vi "SignalMngmnt.vi"(8 "error in (no error)":errorcluster) -> (0 "error out":errorcluster)   [LabVIEW 2012]
uses:
  #TD_SignalStorageCommand.ctl
  #TD_SignalStorageData.ctl
  <vilib>/addons/Wavelet Analysis/typedefs.llb/WA Data.ctl
  <vilib>/Waveform/WDTOps.llb/WDT Get Waveform Subset DBL.vi
  <vilib>/addons/_Advanced Signal Processing/NI_AdvSigProcWA.lvlib
panel:
  in  "CursorReset":bool
  in  "ResetStorage":bool
  in  "Cut":bool
  out "Signal Graph":waveform(dbl)(graph) caption="Podgląd sygnału"
  in  "Signal Description":string caption="Opis sygnału"
  in  "Signal name":string caption="Nazwa sygnału:"
  in  "AddSpecial":bool
  in  "Remove":bool
  in  "Read":bool
  in  "Signal List":i32(listbox) caption="Lista sygnałów"
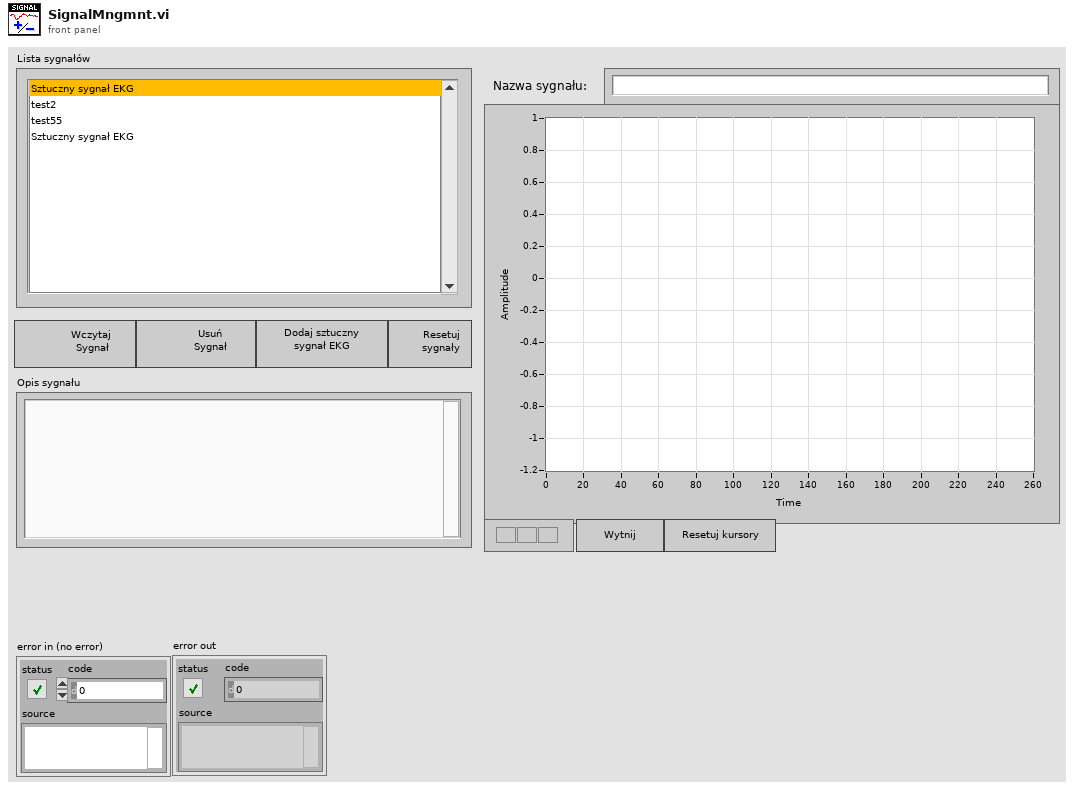
[diagram p1: front panel]
types:
  T1 = cluster{"Signal List":refnum<vi>, "Signal Graph":refnum<vi>, "Signal name":refnum<vi>, "Signal Description":refnum<vi>}
  T2 = typedef "#TD_SignalStorageCommand.ctl" = enum16{"Reset_Storage", "Add_Signal", "Insert_Signal", "Del_Signal", "Replace_Signal", "Get_Signal", "Get_Signal_List", "Change_Signal_Name", "Change_Signal_Descr"}
  T3 = typedef "#TD_SignalStorageData.ctl" = cluster{"Signal":waveform(dbl), "Signal Name":string, "Description":string}
  T4 = typedef "#TD_SignalSpecInfo.ctl" = cluster{"file name":string, "format":i32, "samples per frame":i32, "skew":i32, "byte offset":i32, "ADC gain":dbl, "baseline (ADC units)":i16, "units":string, "ADC resolution":i16, "ADC zero":i16, "initial value":i16, "checksum":i16, "block size":i32, "description":string}
  T5 = typedef "NI_AdvSigProcWA.lvlib/WA Data.ctl" = u16
  T6 = typedef "LVPoint32TypeDef.ctl" = cluster{"Horizontal":i32, "Vertical":i32}
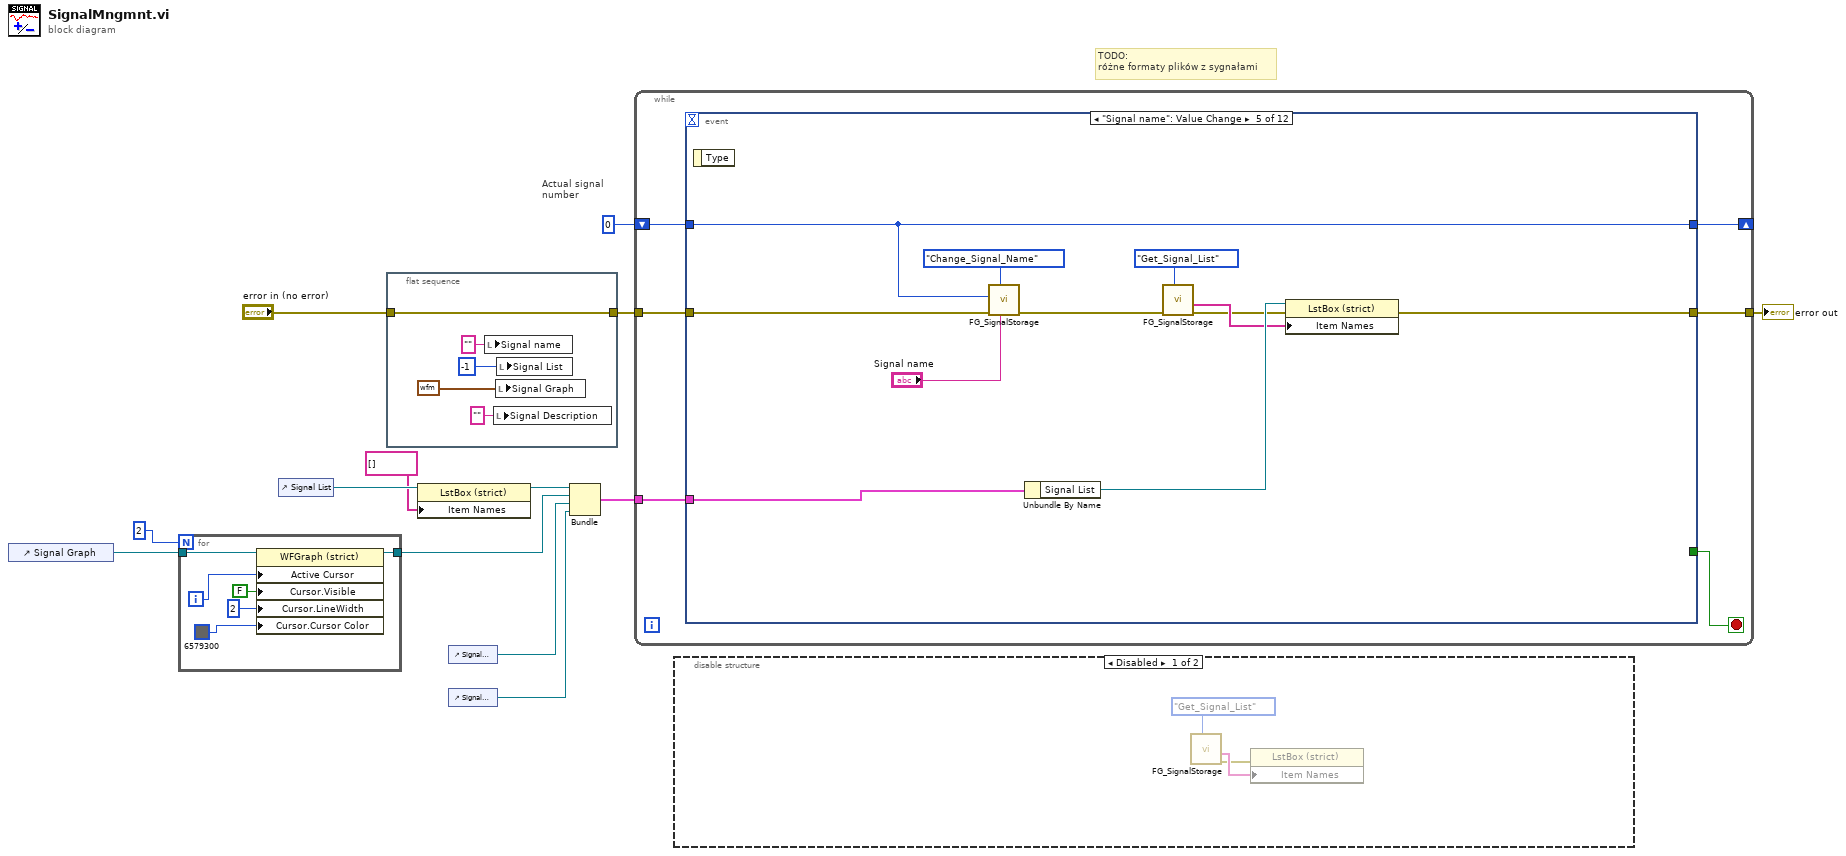
[diagram p0: block diagram]
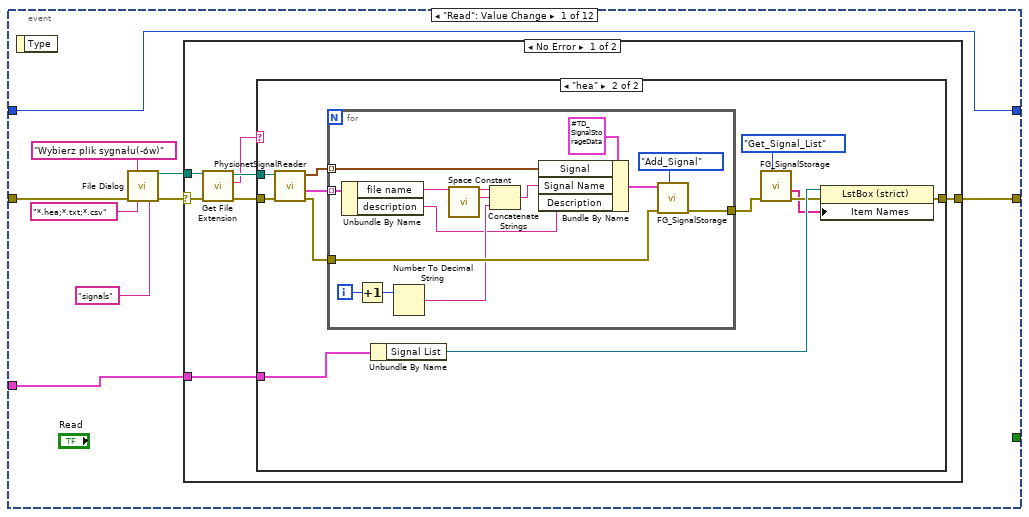
[diagram p3: hidden frame]
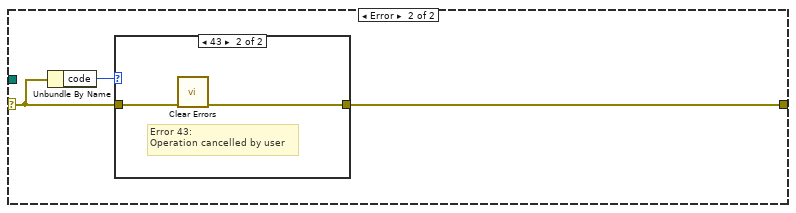
[diagram p5: hidden frame]
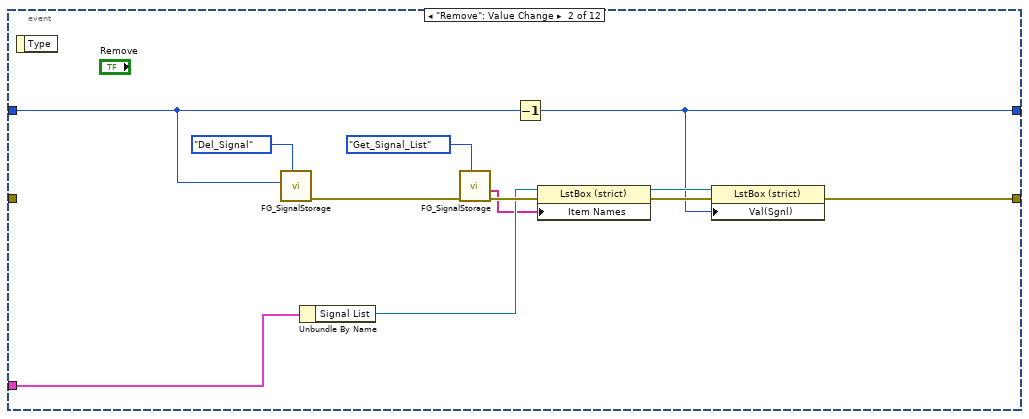
[diagram p7: hidden frame]
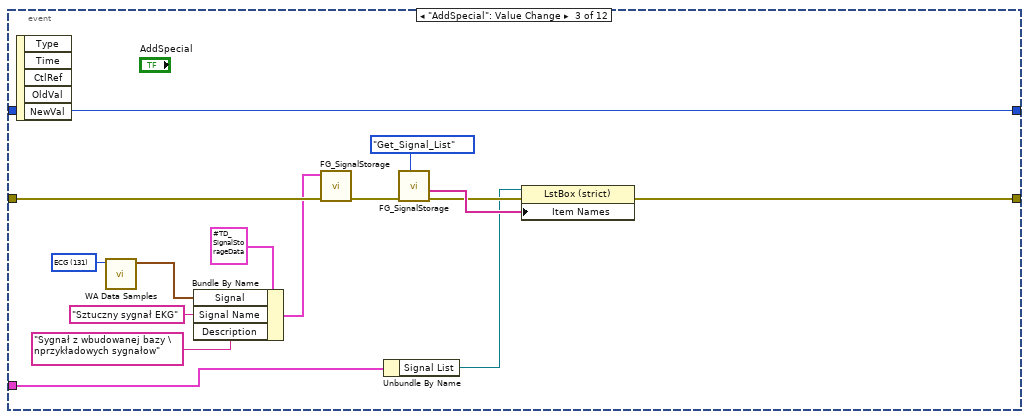
[diagram p8: hidden frame]
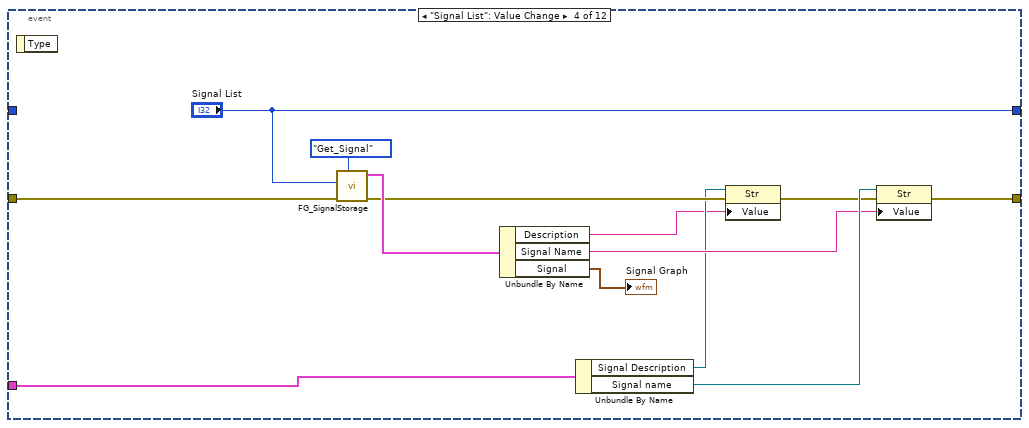
[diagram p9: hidden frame]
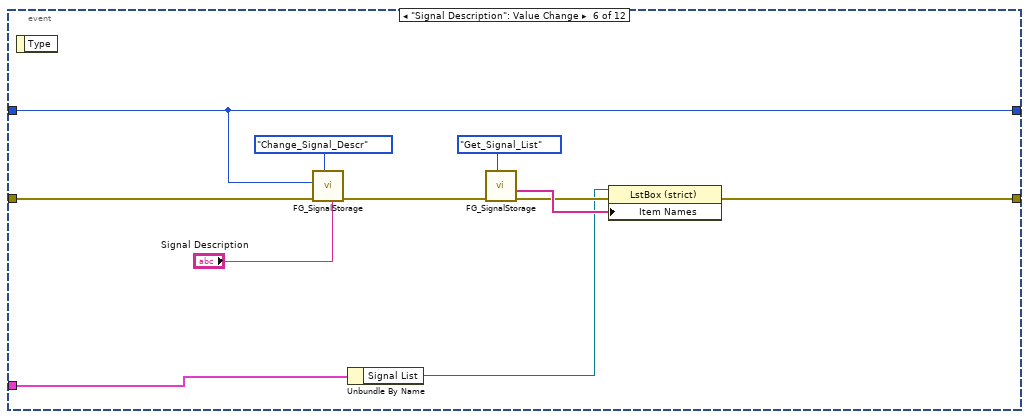
[diagram p10: hidden frame]
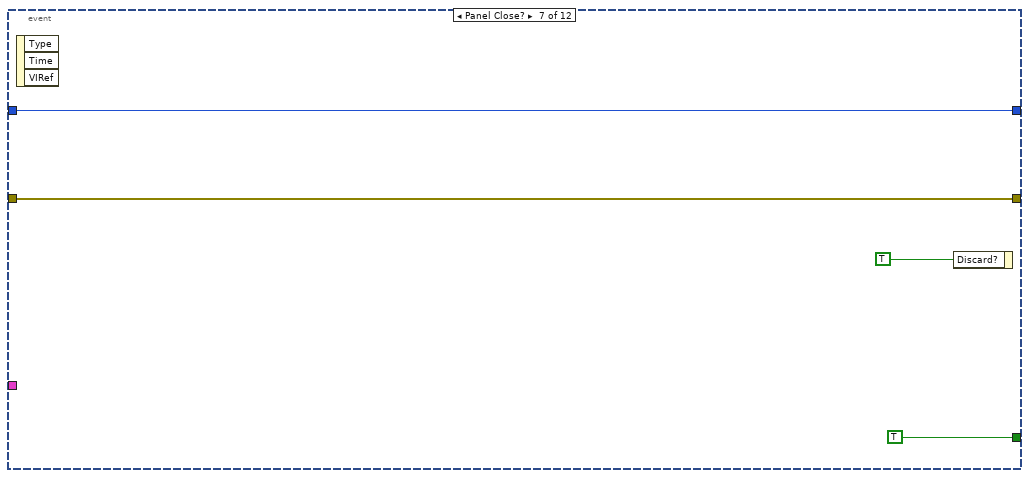
[diagram p11: hidden frame]
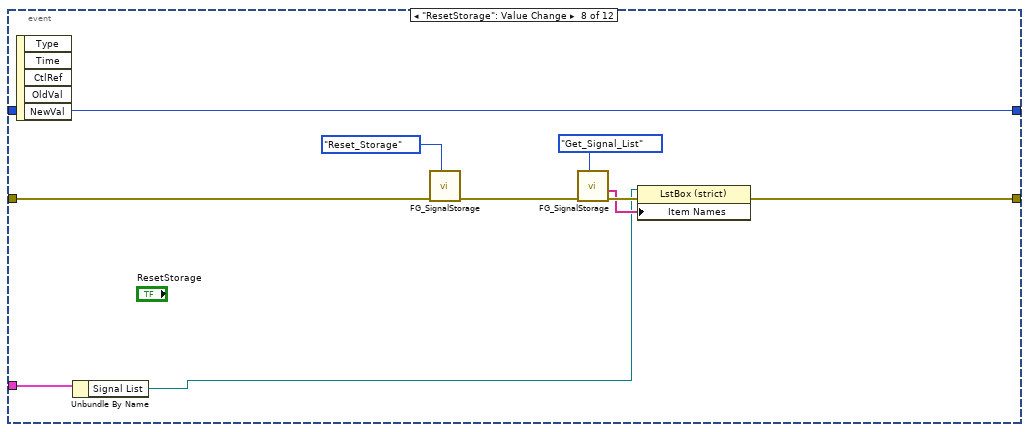
[diagram p12: hidden frame]
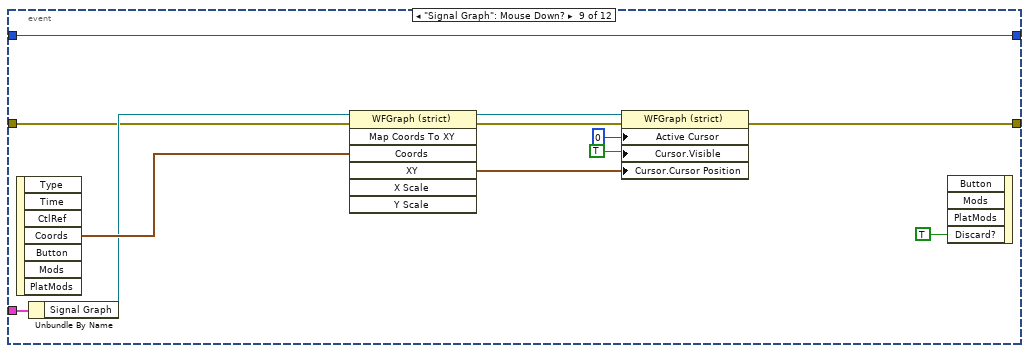
[diagram p13: hidden frame]
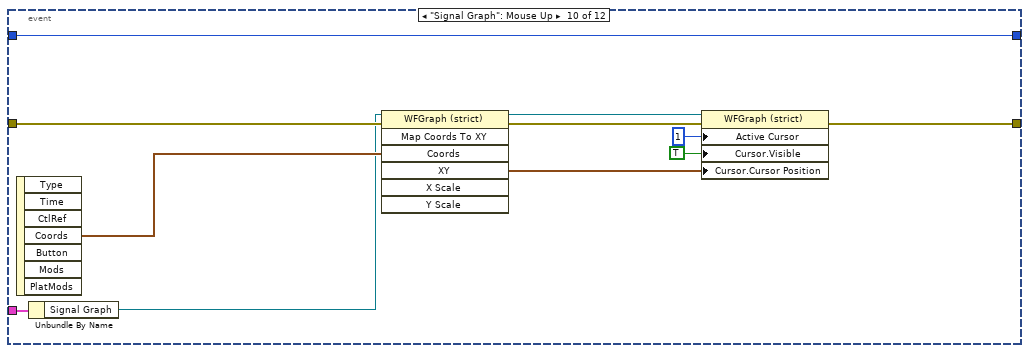
[diagram p14: hidden frame]
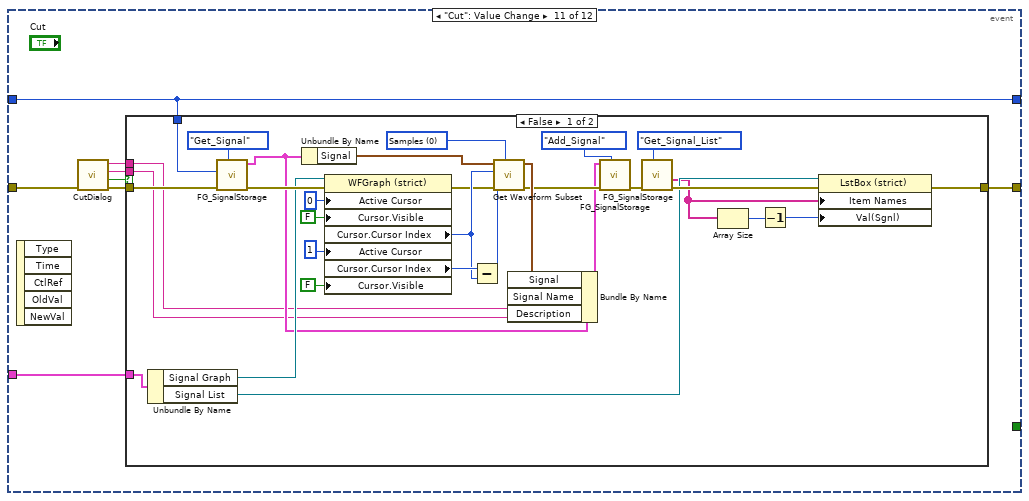
[diagram p15: hidden frame]
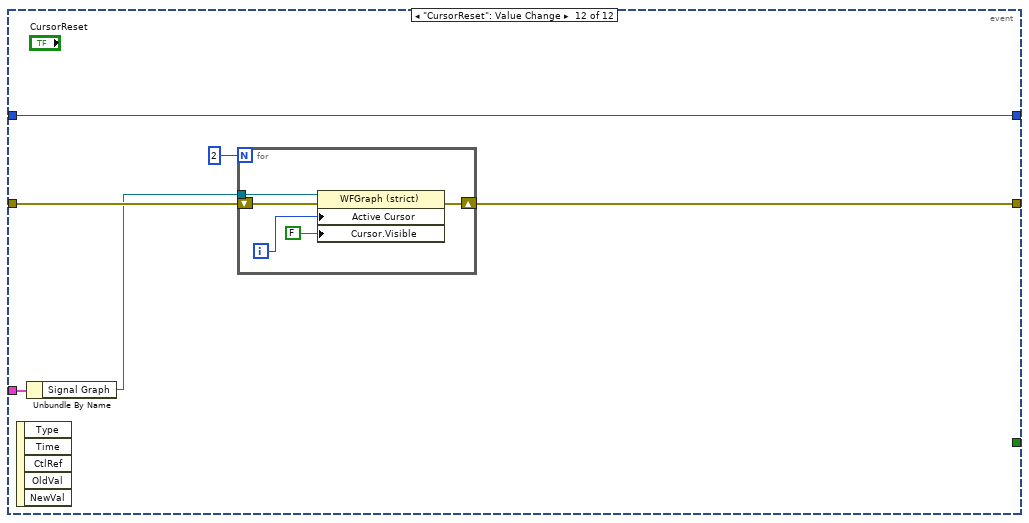
[diagram p17: hidden frame]
diagram:
  # "Actual signal\nnumber"
  # "TODO:\nróżne formaty plików z sygnałami"
  n1 = control-ref of="Signal Graph"() -> (w5:refnum<vi>)
  n2 = for {
    N: 2 -> [_]
    tunnel: w5 -> [w17]
    tunnel: [w16] -> w4
    i -> [w19]
    n3 = property class="WFGraph (strict)"(reference=w17, "Active Cursor"=w19, "Cursor.Visible"=FALSE, "Cursor.LineWidth"=u8 2 ("Cursor.Line Width"), "Cursor.Cursor Color"=u32 6579300) -> (reference out=w16:refnum<vi>)  [unwired: 1 in, 1 out]
  }
  n4 = control-ref of="Signal List"() -> (w11:refnum<vi>)
  n5 = flat-sequence {
    tunnel: [w20] -> w3
    tunnel: "error in (no error)" -> [w20]
    frame #0 {
      n6 = local write "Signal name"("" ("Signal name")) -> ()
      n7 = local write "Signal Description"("" ("Signal Description")) -> ()
      n8 = local write "Signal Graph"(waveform(dbl) {"t0"=timestamp(0 s since 1904-01-01), "dt"=0.0, "Y"=[]} ("Podgląd sygnału")) -> ()
      n9 = local write "Signal List"(-1 ("Lista sygnałów")) -> ()
    }
  }
  n10 = property class="LstBox (strict)"(reference=w11, "Item Names"=string[] []) -> (reference out=w10:refnum<vi>)  [unwired: 1 in, 1 out]
  n11 = control-ref of="Signal name"() -> (w8:refnum<vi>)
  n12 = control-ref of="Signal Description"() -> (w7:refnum<vi>)
  n13 = Bundle("Signal List"=w10, "Signal Graph"=w4, "Signal name"=w8, "Signal Description"=w7) -> (w13:T1)  [unwired: 1 in]
  n14 = while {
    tunnel: [w29] -> w1
    tunnel: w13 -> [w28]
    shift-right: [w26] -> _
    shift-left: 0 ("Lista sygnałów") -> [w27]
    tunnel: w3 -> [w25]
    stop <- w30 stop-if-true
    n15 = event shown="[4] \"Signal name\": Value Change" {
      selector: _ -> [_ _ _ _ _ _ _ _ _ _ _ _]
      dyn-events: _ -> [_ _ _ _ _ _ _ _ _ _ _ _]
      timeout: _ -> [_ _ _ _ _ _ _ _ _ _ _ _]
      tunnel: [_ _ _ _ _ _ TRUE _ _ _ _ _] -> w30
      tunnel: [w34 w83 w96 w112 w127 w133 w142 w148 w156 w168 w181 w220] -> w29
      tunnel: w28 -> [w33 w87 w94 w116 w126 w132 _ w147 w165 w177 w179 w222]
      tunnel: w27 -> [w32 w82 w106 _ w124 w138 w144 w155 w167 w178 w180 w224]
      tunnel: [w32 w80 w106 "Signal List" w124 w138 w144 w155 w167 w178 w180 w224] -> w26
      tunnel: w25 -> [w31 _ w104 w111 w129 w141 w142 w153 w159 w173 w186 w223]
      event "Read": Value Change {
        n16 = event-data() -> ()  [unwired: 1 in, 1 out]
        n17 = call "File Dialog"("prompt"="Wybierz plik sygnału(-ów)", "error in"=w31, "pattern (all files)"="*.hea;*.txt;*.csv", "pattern label"="signals") -> ("selected path"=w37:path, "error out"=w36:errorcluster)  [unwired: 8 in, 2 out]
        n18 = case shown="No Error" w36 {
          selector: w36 -> [w44 w75]
          tunnel: w37 -> [w46 _]
          tunnel: [w41 w74] -> w34
          tunnel: w33 -> [w40 _]
          frame No Error {
            n19 = call <vilib>:"Get File Extension.vi"("error in (no error)"=w44, "file"=w46) -> ("error out"=w43:errorcluster, "lowercase file extension"=w42:string, "dup file"=w45:path)  [unwired: 6 in, 1 out]
            n20 = case shown="\"hea\"" w42 {
              tunnel: w45 -> [_ w57]
              tunnel: w43 -> [w47 w56]
              tunnel: [w47 w49] -> w41
              tunnel: w40 -> [_ w51]
              frame Default {
              }
              frame "hea" {
                n21 = call "PhysionetSignalReader.vi"("error in (no error)"=w56, "Header file path"=w57) -> ("error out"=w55:errorcluster, "Signals Specs Info"=w59:T4[], "Signals(physical units)"=w58:waveform(dbl)[])  [unwired: 5 in, 2 out]
                n22 = for {
                  tunnel: w59 -> [w73] mode=indexing
                  tunnel: w58 -> [w66] mode=indexing
                  tunnel: w55 -> [w64]
                  tunnel: [w63] -> w53
                  i -> [w72]
                  n23 = Unbundle By Name(w73) -> ("file name"=w70:string, "description"=w60:string)
                  n24 = Increment(x=w72) -> (x+1=w71:i32)
                  n25 = Number To Decimal String(number=w71) -> (decimal integer string=w62:string)  [unwired: 1 in]
                  n26 = call <vilib>:"Space Constant.vi"() -> ("String"=w61:string)
                  n27 = Concatenate Strings(w70, w61, w62) -> (w68:string)
                  n28 = Bundle By Name(cluster=T3 {"Signal"={"t0"=timestamp(0 s since 1904-01-01), "dt"=1.0, "Y"=[]}, "Signal Name"="", "Description"=""} ("DataIn"), "Signal"=w66, "Signal Name"=w68, "Description"=w60) -> (w65:T3)
                  n29 = call "FG_SignalStorage.vi"("Command"=#TD_SignalStorageCommand."Add_Signal", "error in (no error)"=w64, "DataIn"=w65) -> ("error out"=w63:errorcluster)  [unwired: 6 in, 2 out]
                }
                n30 = Unbundle By Name(w51) -> ("Signal List"=w52:refnum<vi>)
                n31 = call "FG_SignalStorage.vi"("Command"=#TD_SignalStorageCommand."Get_Signal_List", "error in (no error)"=w53) -> ("error out"=w50:errorcluster, "Signal_List"=w48:string[])  [unwired: 7 in, 1 out]
                n32 = property class="LstBox (strict)"(reference=w52, error in=w50, "Item Names"=w48) -> (error out=w49:errorcluster)  [unwired: 1 out]
              }
            }
          }
          frame Error {
            n33 = Unbundle By Name(w75) -> ("code"=w76:i32)
            n34 = case shown="43" w76 {
              tunnel: w75 -> [w77 w79]
              tunnel: [w77 w78] -> w74
              frame Default {
              }
              frame 43 {
                # "Error 43: \nOperation cancelled by user"
                n35 = call <vilib>:"Clear Errors.vi"("error in (no error)"=w79) -> ("error out"=w78:errorcluster)  [unwired: 6 in]
              }
            }
          }
        }
      }
      event "Remove": Value Change {
        n36 = event-data() -> ()  [unwired: 1 in, 1 out]
        n37 = call "FG_SignalStorage.vi"("Command"=#TD_SignalStorageCommand."Del_Signal", "SignalNumber"=w82) -> ("error out"=w88:errorcluster)  [unwired: 7 in, 2 out]
        n38 = Unbundle By Name(w87) -> ("Signal List"=w86:refnum<vi>)
        n39 = call "FG_SignalStorage.vi"("Command"=#TD_SignalStorageCommand."Get_Signal_List", "error in (no error)"=w88) -> ("error out"=w90:errorcluster, "Signal_List"=w81:string[])  [unwired: 7 in, 1 out]
        n40 = Decrement(x=w82) -> (x-1=w80:i32)
        n41 = property class="LstBox (strict)"(reference=w86, error in=w90, "Item Names"=w81) -> (reference out=w84:refnum<vi>, error out=w85:errorcluster)
        n42 = property class="LstBox (strict)"(reference=w84, error in=w85, "Val(Sgnl)"=w80) -> (error out=w83:errorcluster)  [unwired: 1 out]
      }
      event "AddSpecial": Value Change {
        w105 = T5 131 items=["1D Example Data"=100, "-"=101, "Doppler"=102, "HOP"=103, "TF Sine"=104, "Noisy Doppler"=105, "Sea Temperature"=106, "Sp500"=107, "Power Line"=108, "Engine Knocking"=109, "HeaviSine"=110, "Bumps"=111, "Blocks"=112, "Piece Regular"=113, "HypChirps"=114, "LinChirps"=115, "Chirps"=116, "Piece Polynomial"=117, "ECG"=131, "-"=118, "2D Example Data"=119, "-"=120, "Finger Print (Image)"=121, "Iris Flower (Image)"=122, "Mammogram (Image)"=123, "Lake (Image)"=127, "Two Can 1 (Image)"=132, "Two Can 2 (Image)"=133, "Camera Man (Image)"=134] ("data")
        n43 = event-data() -> ()  [unwired: 1 in, 5 out]
        n44 = call <vilib>:"WA Data Samples.vi"("data"=w105) -> ("signal"=w102:waveform(dbl))  [unwired: 9 in, 1 out]
        n45 = Bundle By Name(cluster=T3 {"Signal"={"t0"=timestamp(0 s since 1904-01-01), "dt"=1.0, "Y"=[]}, "Signal Name"="", "Description"=""} ("DataIn"), "Signal"=w102, "Signal Name"="Sztuczny sygnał EKG", "Description"="Sygnał z wbudowanej bazy \nprzykładowych sygnałow") -> (w101:T3)
        n46 = call "FG_SignalStorage.vi"("error in (no error)"=w104, "DataIn"=w101) -> ("error out"=w97:errorcluster)  [unwired: 7 in, 2 out]
        n47 = Unbundle By Name(w94) -> ("Signal List"=w93:refnum<vi>)
        n48 = call "FG_SignalStorage.vi"("Command"=#TD_SignalStorageCommand."Get_Signal_List", "error in (no error)"=w97) -> ("error out"=w98:errorcluster, "Signal_List"=w99:string[])  [unwired: 7 in, 1 out]
        n49 = property class="LstBox (strict)"(reference=w93, error in=w98, "Item Names"=w99) -> (error out=w96:errorcluster)  [unwired: 1 out]
      }
      event "Signal List": Value Change {
        n50 = event-data() -> ()  [unwired: 1 in, 1 out]
        n51 = call "FG_SignalStorage.vi"("Command"=#TD_SignalStorageCommand."Get_Signal", "error in (no error)"=w111, "SignalNumber"="Signal List") -> ("error out"=w110:errorcluster, "DataOut"=w117:T3)  [unwired: 6 in, 1 out]
        n52 = Unbundle By Name(w117) -> ("Description"=w107:string, "Signal Name"=w114:string, "Signal"=→"Signal Graph":waveform(dbl))
        n53 = Unbundle By Name(w116) -> ("Signal Description"=w109:refnum<vi>, "Signal name"=w115:refnum<vi>)
        n54 = property class="Str"(reference=w109, error in=w110, "Value"=w107) -> (error out=w108:errorcluster)  [unwired: 1 out]
        n55 = property class="Str"(reference=w115, error in=w108, "Value"=w114) -> (error out=w112:errorcluster)  [unwired: 1 out]
      }
      event "Signal name": Value Change {
        n56 = event-data() -> ()  [unwired: 1 in, 1 out]
        n57 = call "FG_SignalStorage.vi"("Signal Name"="Signal name", "Command"=#TD_SignalStorageCommand."Change_Signal_Name", "error in (no error)"=w129, "SignalNumber"=w124) -> ("error out"=w123:errorcluster)  [unwired: 5 in, 2 out]
        n58 = Unbundle By Name(w126) -> ("Signal List"=w125:refnum<vi>)
        n59 = call "FG_SignalStorage.vi"("Command"=#TD_SignalStorageCommand."Get_Signal_List", "error in (no error)"=w123) -> ("error out"=w120:errorcluster, "Signal_List"=w121:string[])  [unwired: 7 in, 1 out]
        n60 = property class="LstBox (strict)"(reference=w125, error in=w120, "Item Names"=w121) -> (error out=w127:errorcluster)  [unwired: 1 out]
      }
      event "Signal Description": Value Change {
        n61 = event-data() -> ()  [unwired: 1 in, 1 out]
        n62 = call "FG_SignalStorage.vi"("Signal Descr."="Signal Description", "Command"=#TD_SignalStorageCommand."Change_Signal_Descr", "error in (no error)"=w141, "SignalNumber"=w138) -> ("error out"=w134:errorcluster)  [unwired: 5 in, 2 out]
        n63 = Unbundle By Name(w132) -> ("Signal List"=w131:refnum<vi>)
        n64 = call "FG_SignalStorage.vi"("Command"=#TD_SignalStorageCommand."Get_Signal_List", "error in (no error)"=w134) -> ("error out"=w135:errorcluster, "Signal_List"=w136:string[])  [unwired: 7 in, 1 out]
        n65 = property class="LstBox (strict)"(reference=w131, error in=w135, "Item Names"=w136) -> (error out=w133:errorcluster)  [unwired: 1 out]
      }
      event Panel Close? {
        n66 = event-data() -> ()  [unwired: 1 in, 3 out]
        n67 = event-data("Discard?"=TRUE) -> ()  [unwired: 1 in, 1 out]
      }
      event "ResetStorage": Value Change {
        n68 = event-data() -> ()  [unwired: 1 in, 5 out]
        n69 = Unbundle By Name(w147) -> ("Signal List"=w146:refnum<vi>)
        n70 = call "FG_SignalStorage.vi"("Command"=#TD_SignalStorageCommand."Reset_Storage", "error in (no error)"=w153) -> ("error out"=w149:errorcluster)  [unwired: 7 in, 2 out]
        n71 = call "FG_SignalStorage.vi"("Command"=#TD_SignalStorageCommand."Get_Signal_List", "error in (no error)"=w149) -> ("error out"=w151:errorcluster, "Signal_List"=w150:string[])  [unwired: 7 in, 1 out]
        n72 = property class="LstBox (strict)"(reference=w146, error in=w151, "Item Names"=w150) -> (error out=w148:errorcluster)  [unwired: 1 out]
      }
      event "Signal Graph": Mouse Down? {
        n73 = event-data() -> ("Coords"=w162:T6)  [unwired: 1 in, 6 out]
        n74 = Unbundle By Name(w165) -> ("Signal Graph"=w161:refnum<vi>)
        n75 = invoke class="WFGraph (strict)" method="Map Coords To XY"(reference=w161, error in=w159, "Coords"=w162) -> (reference out=w160:refnum<vi>, error out=w158:errorcluster, "XY"=w157:cluster{"X":dbl, "Y":dbl})  [unwired: 4 in, 4 out]
        n76 = property class="WFGraph (strict)"(reference=w160, error in=w158, "Active Cursor"=u32 0, "Cursor.Visible"=TRUE, "Cursor.Cursor Position"=w157) -> (error out=w156:errorcluster)  [unwired: 1 out]
        n77 = event-data("Discard?"=TRUE) -> ()  [unwired: 4 in, 1 out]
      }
      event "Signal Graph": Mouse Up {
        n78 = event-data() -> ("Coords"=w174:T6)  [unwired: 1 in, 6 out]
        n79 = Unbundle By Name(w177) -> ("Signal Graph"=w170:refnum<vi>)
        n80 = invoke class="WFGraph (strict)" method="Map Coords To XY"(reference=w170, error in=w173, "Coords"=w174) -> (reference out=w169:refnum<vi>, error out=w171:errorcluster, "XY"=w172:cluster{"X":dbl, "Y":dbl})  [unwired: 4 in, 4 out]
        n81 = property class="WFGraph (strict)"(reference=w169, error in=w171, "Active Cursor"=u32 1, "Cursor.Visible"=TRUE, "Cursor.Cursor Position"=w172) -> (error out=w168:errorcluster)  [unwired: 1 out]
      }
      event "Cut": Value Change {
        n82 = event-data() -> ()  [unwired: 1 in, 5 out]
        n83 = call "CutDialog.vi"("error in (no error)"=w186) -> ("error out"=w184:errorcluster, "Cancelled"=w185:bool, "CommentOut"=w183:string, "NameOut"=w182:string)  [unwired: 7 in]
        n84 = case shown="False" w185 {
          tunnel: w184 -> [w217 w218]
          tunnel: w183 -> [w200 _]
          tunnel: w182 -> [w201 _]
          tunnel: [w187 w218] -> w181
          tunnel: w180 -> [w216 _]
          tunnel: w179 -> [w213 _]
          frame False {
            w209 = u16 0 items=["Samples", "Relative Time"] ("start/duration format")
            n85 = Unbundle By Name(w213) -> ("Signal Graph"=w212:refnum<vi>, "Signal List"=w193:refnum<vi>)
            n86 = call "FG_SignalStorage.vi"("Command"=#TD_SignalStorageCommand."Get_Signal", "error in (no error)"=w217, "SignalNumber"=w216) -> ("error out"=w214:errorcluster, "DataOut"=w203:T3)  [unwired: 6 in, 1 out]
            n87 = Unbundle By Name(w203) -> ("Signal"=w208:waveform(dbl))
            n88 = property class="WFGraph (strict)"(reference=w212, error in=w214, "Active Cursor"=u32 0, "Cursor.Visible"=FALSE, "Active Cursor"=u32 1, "Cursor.Visible"=FALSE) -> (error out=w204:errorcluster, "Cursor.Cursor Index"=w206:i32, "Cursor.Cursor Index"=w207:i32)  [unwired: 1 out]
            n89 = Subtract(x=w207, y=w206) -> (x-y=w205:i32)
            n90 = call-poly <vilib>:"Get Waveform Subset.vi"("start/duration format"=w209, "error in (no error)"=w204, "duration"=w205, "start samples/time"=w206, "waveform in"=w208) -> ("error out"=w198:errorcluster, "waveform out"=w202:waveform(dbl))  [unwired: 1 in, 2 out]
            n91 = Bundle By Name(cluster=w203, "Signal"=w202, "Signal Name"=w201, "Description"=w200) -> (w197:T3)
            n92 = call "FG_SignalStorage.vi"("Command"=#TD_SignalStorageCommand."Add_Signal", "error in (no error)"=w198, "DataIn"=w197) -> ("error out"=w194:errorcluster)  [unwired: 6 in, 2 out]
            n93 = call "FG_SignalStorage.vi"("Command"=#TD_SignalStorageCommand."Get_Signal_List", "error in (no error)"=w194) -> ("error out"=w195:errorcluster, "Signal_List"=w190:string[])  [unwired: 7 in, 1 out]
            n94 = Array Size(array=w190) -> (size(s)=w189:i32)
            n95 = Decrement(x=w189) -> (x-1=w188:i32)
            n96 = property class="LstBox (strict)"(reference=w193, error in=w195, "Item Names"=w190, "Val(Sgnl)"=w188) -> (error out=w187:errorcluster)  [unwired: 1 out]
          }
          frame True {
            # "Cancelled"
          }
        }
      }
      event "CursorReset": Value Change {
        n97 = event-data() -> ()  [unwired: 1 in, 5 out]
        n98 = Unbundle By Name(w222) -> ("Signal Graph"=w221:refnum<vi>)
        n99 = for {
          N: 2 -> [_]
          tunnel: w221 -> [w228]
          shift-right: [w225] -> w220
          shift-left: w223 -> [w229]
          i -> [w226]
          n100 = property class="WFGraph (strict)"(reference=w228, error in=w229, "Active Cursor"=w226, "Cursor.Visible"=FALSE) -> (error out=w225:errorcluster)  [unwired: 1 out]
        }
      }
    }
  }
  "error out" <- w1
  n101 = disable-structure shown="Disabled" {
    frame Disabled {
      n102 = call "FG_SignalStorage.vi"("Command"=#TD_SignalStorageCommand."Get_Signal_List") -> ("error out"=w231:errorcluster, "Signal_List"=w232:string[])  [unwired: 8 in, 1 out]
      n103 = property class="LstBox (strict)"(error in=w231, "Item Names"=w232) -> ()  [unwired: 1 in, 2 out]
    }
    frame Enabled {
    }
  }
